vi "Analog Input - Vibration.vi"(5 "Samples to Read":i32=2560, 7 "Action":enum16{"Initialize", "Read", "Close"}(ring), 8 "error in (no error)":errorcluster, 9 "Sample Rate":dbl=25600.0, 10 "Channel":tag="Mod1/ai0", 11 "task in":refnum<k21>) -> (0 "error out":errorcluster, 2 "data":waveform(dbl), 3 "task out":refnum<k21>)   [LabVIEW 2017]
uses:
  <vilib>/DAQmx/read.llb/DAQmx Read (Analog Wfm 1Chan NSamp).vi
  <vilib>/DAQmx/create/channels.llb/DAQmx Create Channel (AI-Voltage-Basic).vi
  <vilib>/DAQmx/configure/timing.llb/DAQmx Timing (Sample Clock).vi
  <vilib>/DAQmx/miscellaneous.llb/DAQmx Fill In Error Info.vi
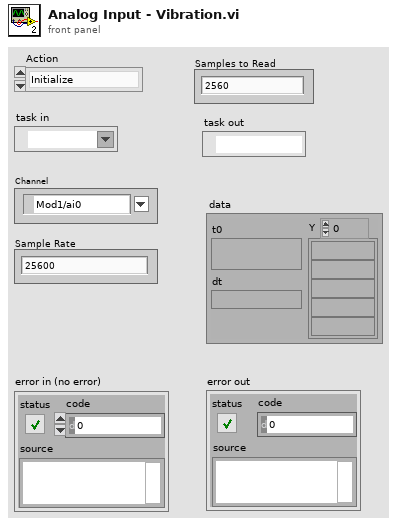
[diagram p1: front panel]
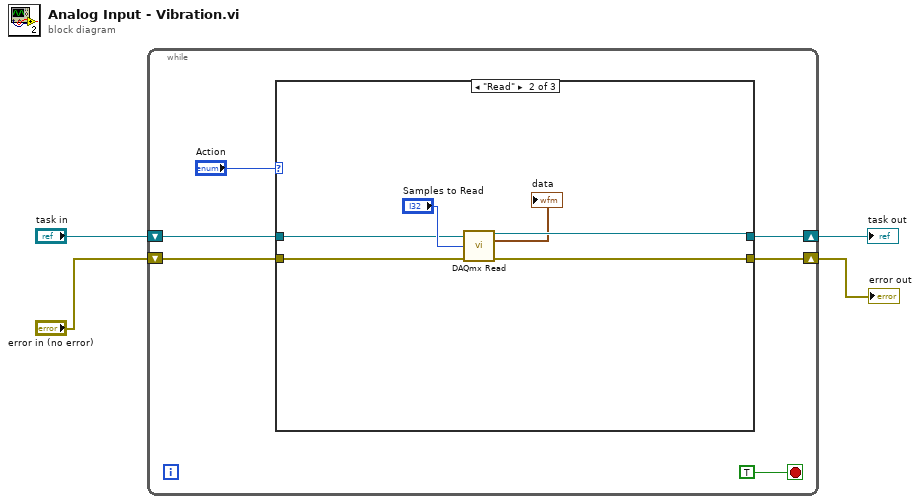
[diagram p0: block diagram]
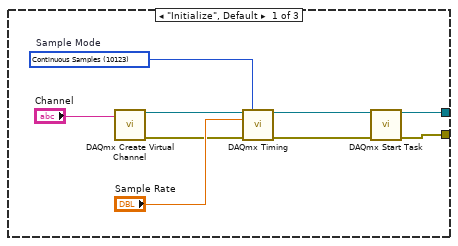
[diagram p2: hidden frame]
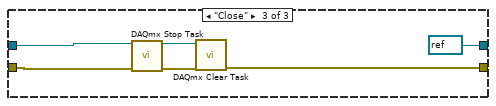
[diagram p3: hidden frame]
diagram:
  n1 = while {
    shift-right: [w8] -> w3
    shift-left: "task in" -> [w7]
    shift-right: [w5] -> w4
    shift-left: "error in (no error)" -> [w6]
    stop <- TRUE stop-if-true
    n2 = case shown="\"Read\"" "Action" {
      tunnel: [w12 w22 refnum<k21> refnum ("task out")] -> w8
      tunnel: [w11 w24 w27] -> w5
      tunnel: w7 -> [_ w23 w29]
      tunnel: w6 -> [_ w21 w28]
      frame "Initialize", Default {
        w17 = 10123 items=["Finite Samples"=10178, "Continuous Samples"=10123, "Hardware Timed Single Point"=12522]  # Sample Mode
        n3 = call-poly <vilib>:"DAQmx Create Virtual Channel.vi"("physical channels"="Channel") -> ("task out"=w14:refnum<k21>, "error out"=w15:errorcluster)  [unwired: 13 in]
        n4 = call-poly <vilib>:"DAQmx Timing.vi"("task/channels in"=w14, "sample mode"=w17, "rate"="Sample Rate", "error in"=w15) -> ("task out"=w19:refnum<k21>, "error out"=w18:errorcluster)  [unwired: 10 in]
        n5 = call <vilib>:"DAQmx Start Task.vi"("task/channels in"=w19, "error in"=w18) -> ("task out"=w12:refnum<k21>, "error out"=w11:errorcluster)  [unwired: 12 in]
      }
      frame "Read" {
        n6 = call-poly <vilib>:"DAQmx Read.vi"("task/channels in"=w23, "number of samples per channel"="Samples to Read", "error in"=w21) -> ("task out"=w22:refnum<k21>, "data"=→"data":waveform(dbl), "error out"=w24:errorcluster)  [unwired: 10 in]
      }
      frame "Close" {
        n7 = call <vilib>:"DAQmx Stop Task.vi"("task/channels in"=w29, "error in"=w28) -> ("task out"=w30:refnum<k21>, "error out"=w31:errorcluster)  [unwired: 12 in]
        n8 = call <vilib>:"DAQmx Clear Task.vi"("task in"=w30, "error in"=w31) -> ("error out"=w27:errorcluster)  [unwired: 13 in]
      }
    }
  }
  "error out" <- w4
  "task out" <- w3
